vi "Set Frequency.vi"(8 "error in (no error)":errorcluster, 9 "frequency":dbl[unit], 10 "Channel (0: Channel 1)":T1 items=["Channel 1", "Channel 2"], 11 "VISA resource name":refnum<visa-resource-name>) -> (0 "error out":errorcluster, 3 "VISA resource name out":refnum<visa-resource-name>)   [LabVIEW 2017, in "Tektronix AFG 3000 Series.lvlib"]
doc: "Sets the frequency of a Tektronix AFG 3000 series function generator. May not be used when the run mode is set to sweep. Note: if you change the output waveform, this frequency may change, since the range of frequencies available will be different."
uses:
  Tektronix AFG 3000 Series.lvlib
  controls.llb/Channel.ctl
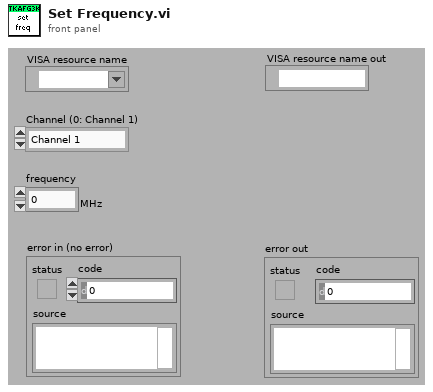
[diagram p1: front panel]
types:
  T1 = typedef "Channel.ctl" = u16
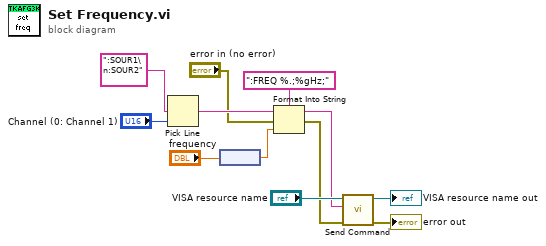
[diagram p0: block diagram]
diagram:
  n1 = Pick Line(multi-line string=":SOUR1\n:SOUR2", line index="Channel (0: Channel 1)") -> (output string=w9:string)  [unwired: 1 out]
  n2 = node("frequency") -> (w6:dbl)
  n3 = Format Into String(format string=":FREQ %.;%gHz;", initial string=w9, error in="error in (no error)", w6) -> (resulting string=w5:string, error out=w3:errorcluster)
  n4 = call "Send Command.vi"("error in (no error)"=w3, "write buffer"=w5, "VISA resource name"="VISA resource name") -> ("error out"=→"error out":errorcluster, "VISA resource name out"=→"VISA resource name out":refnum<visa-resource-name>)  [unwired: 7 out]
